vi "mode converting.vi"(11 "IOName输入":refnum<vi>) -> (0 "错误输出":errorcluster, 3 "引用句柄输出":refnum<k21>)   [LabVIEW 2017]
uses:
  <vilib>/VirtualBench/VirtualBench.lvlib
panel:
  in  "Data":bool[](array[boolean])=[TRUE, FALSE]
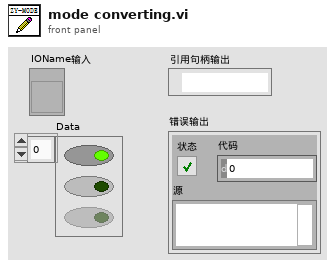
[diagram p1: front panel]
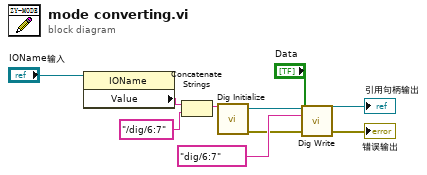
[diagram p0: block diagram]
diagram:
  n1 = property class="IOName"(reference="IOName输入") -> ("Value"=w9:string)  [unwired: 1 in, 2 out]
  n2 = Concatenate Strings(w9, "/dig/6:7" ("字符串")) -> (w3:string)
  n3 = call <vilib>:"Dig Initialize.vi"("Lines"=w3) -> ("Instrument Handle Out"=w6:refnum<k21>, "Error Out"=w4:errorcluster)  [unwired: 13 in]
  n4 = call <vilib>:"Dig Write.vi"("Instrument Handle In"=w6, "Lines"=tag "dig/6:7", "Data"="Data", "Error In"=w4) -> ("Instrument Handle Out"=→"引用句柄输出":refnum<k21>, "Error Out"=→"错误输出":errorcluster)  [unwired: 10 in]
